vi "waveform_conversion.vi"(10 "sample length":i32, 11 "Array":waveform(dbl)[](array[waveform])) -> (3 "mean":dbl)   [LabVIEW 2026]
uses:
  <vilib>/ptbypt/NI_PtbyPt.lvlib
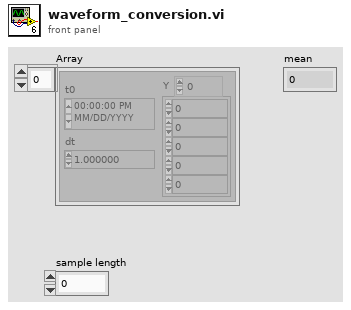
[diagram p1: front panel]
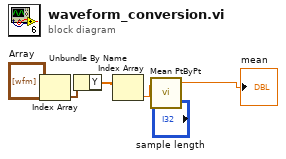
[diagram p0: block diagram]
diagram:
  n1 = Index Array(array="Array") -> (element=w2:waveform(dbl))  [unwired: 1 in]
  n2 = Unbundle By Name(w2) -> ("Y"=w4:dbl[])
  n3 = Index Array(array=w4) -> (element=w5:dbl)  [unwired: 1 in]
  n4 = call <vilib>:"Mean PtByPt.vi"("x"=w5, "sample length"="sample length") -> ("mean"=→"mean":dbl)  [unwired: 2 in, 1 out]
